vi "檢測_距離clamp_VI.vi"(7 "setting":T1={"Contrast"=40, "Filter width"=4, "Steepness"=2, "Subsampling Ratio"=5}, 8 "error in (no error)":errorcluster, 9 "Coordinate System":T2 {"Measurement System"."Axis Reference" items=["Direct", "Indirect"]; "Measurement System"."Angle (deg)" format="%.2f"; "Measurement System"."Origin"."Y" format="%.2f"; "Measurement System"."Origin"."X" format="%.2f"; "Reference System"."Axis Reference" items=["Direct", "Indirect"]; "Reference System"."Angle (deg)" format="%.2f"; "Reference System"."Origin"."Y" format="%.2f"; "Reference System"."Origin"."X" format="%.2f"}, 10 "ROI Descriptor":T4 {"Contours"."Type" items=["No Selection", "Point", "Line", "Rectangle", "Oval", "Polygon", "Freehand Region", "Annulus", "Unused2", "Unused3", "Broken Line", "Freehand Line", "Rotated Rectangle"]}, 11 "Image":T3) -> (0 "error out":errorcluster, 1 "Coordinate System (duplicate)":T2 {"Measurement System"."Axis Reference" items=["Direct", "Indirect"]; "Measurement System"."Angle (deg)" format="%.2f"; "Measurement System"."Origin"."Y" format="%.2f"; "Measurement System"."Origin"."X" format="%.2f"; "Reference System"."Axis Reference" items=["Direct", "Indirect"]; "Reference System"."Angle (deg)" format="%.2f"; "Reference System"."Origin"."Y" format="%.2f"; "Reference System"."Origin"."X" format="%.2f"}, 2 "Distance":sgl format="%.2f", 3 "Image Out":T3)   [LabVIEW 2015]
uses:
  <vilib>/vision/Image Controls.llb/IMAQ Image.ctl
  <vilib>/vision/NI_Vision_Development_Module.lvlib
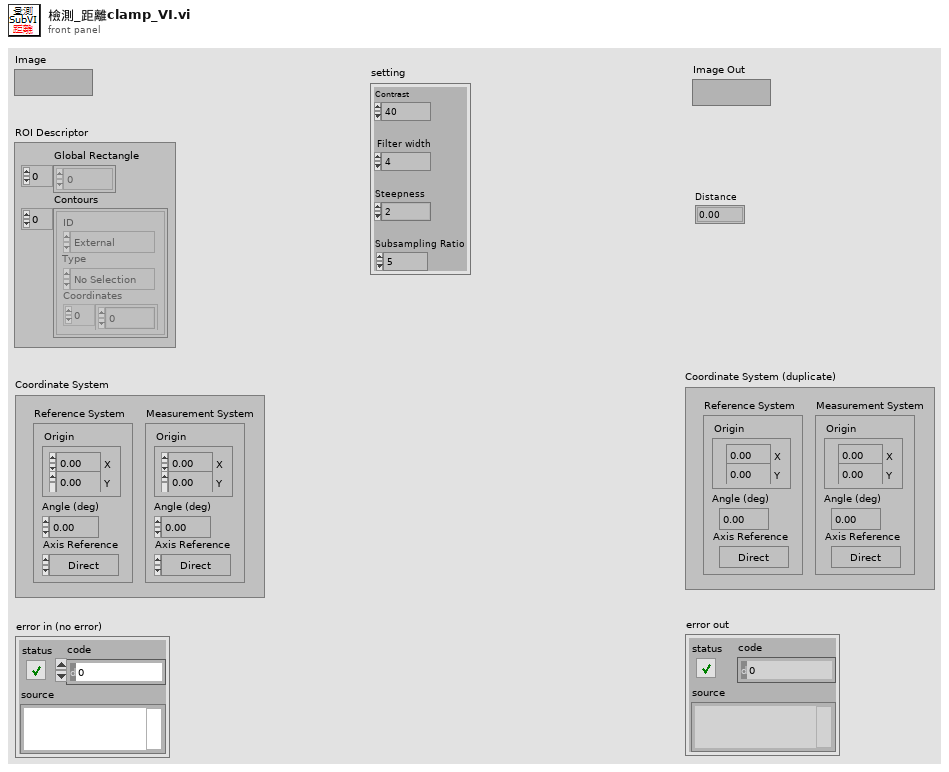
[diagram p1: front panel]
types:
  T1 = cluster{"Contrast":i32, "Filter width":i32, "Steepness":i32, "Subsampling Ratio":u32}
  T2 = typedef "IMAQ Coordinate System" = cluster{"Reference System":cluster{"Origin":cluster{"X":sgl, "Y":sgl}, "Angle (deg)":sgl, "Axis Reference":u32}, "Measurement System":cluster{"Origin":cluster{"X":sgl, "Y":sgl}, "Angle (deg)":sgl, "Axis Reference":u32}}
  T3 = typedef "IMAQ Image.ctl" = refnum<image>
  T4 = typedef "ROI Descriptor" = cluster{"Global Rectangle":i32[], "Contours":cluster{"ID":enum32{"External", "Internal"}, "Type":u32, "Coordinates":i32[]}[]}
  T5 = cluster{"Contrast":i32, "Filter width":i32, "Steepness":i32, "Subsampling Ratio":u32, "Show Search Area":bool, "Show Search Lines":bool, "Show Edges Found":bool, "Show Result":bool}
  T6 = typedef "IMAQ Rectangle" = cluster{"Left":i32, "Top":i32, "Right":i32, "Bottom":i32, "Rotation":dbl}
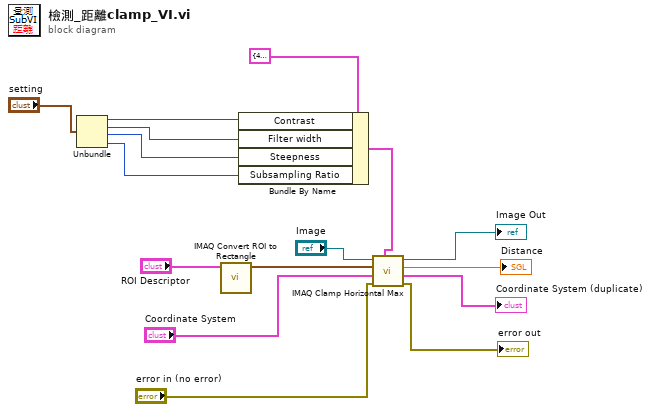
[diagram p0: block diagram]
diagram:
  n1 = Unbundle("setting") -> ("Contrast"=w4:i32, "Filter width"=w3:i32, "Steepness"=w2:i32, "Subsampling Ratio"=w1:u32)
  n2 = call "IMAQ Convert ROI to Rectangle"("ROI Descriptor"="ROI Descriptor") -> ("Rectangle"=w15:T6)  [unwired: 8 in, 1 out]
  n3 = Bundle By Name(cluster=T5 {"Contrast"=40, "Filter width"=4, "Steepness"=2, "Subsampling Ratio"=5, "Show Search Area"=FALSE, "Show Search Lines"=FALSE, "Show Edges Found"=TRUE, "Show Result"=TRUE} ("Settings"), "Contrast"=w4, "Filter width"=w3, "Steepness"=w2, "Subsampling Ratio"=w1) -> (w6:T5)
  n4 = call "IMAQ Clamp Horizontal Max"("Settings"=w6, "error in (no error)"="error in (no error)", "Coordinate System"="Coordinate System", "Rectangle"=w15, "Image"="Image") -> ("error out"=→"error out":errorcluster, "Coordinate System (duplicate)"=→"Coordinate System (duplicate)":T2, "Distance"=→"Distance":sgl, "Image Out"=→"Image Out":T3)  [unwired: 2 in, 1 out]
